vi "Find Zombies.vi"(8 "Error In":errorcluster) -> (0 "Error Out":errorcluster)   [LabVIEW 2018, in "Tests.lvlib" / "Toolkit.lvlib"]
uses:
  Toolkit.lvlib
  <vilib>/addons/_JKI Toolkits/Caraya/classes/Test/Test.lvclass
  <vilib>/addons/_JKI Toolkits/Caraya/classes/Assert/Assert.lvclass
  src/Toolkit/Toolkit.lvlib
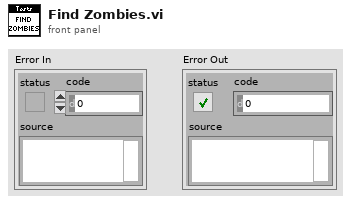
[diagram p1: front panel]
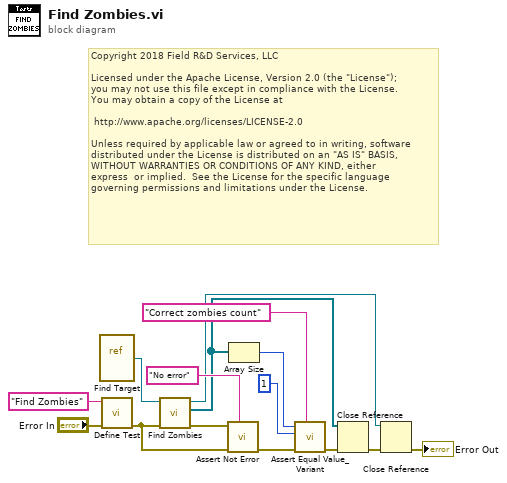
[diagram p0: block diagram]
diagram:
  # "Copyright 2018 Field R&D Services, LLC\n\nLicensed under the Apache License, Version 2.0 (the \"License\");\nyou may not use this file except in compliance with the License.\nYou may obtain a copy of the License at\n\n\thttp://www.apache.org/licenses/LICENSE-2.0\n\nUnless required by applicable law or agreed to in writing, software\ndistributed under the License is distributed on an \"AS IS\" BASIS,\nWITHOUT WARRANTIES OR CONDITIONS OF ANY KIND, either \nexpress  or implied.  See the License for the specific language \ngoverning permissions and limitations under the License."
  n1 = vi-ref "Find Target.vi"() -> (w6:refnum<vi>)
  n2 = call <vilib>:"Define Test.vi"("error in (no error)"="Error In", "Label (VI Title)"="Find Zombies") -> ("error out"=w5:errorcluster)  [unwired: 9 in]
  n3 = call "Find Zombies.vi"("Error In"=w5, "VI In"=w6) -> ("Error Out"=w15:errorcluster, "Graves"=w3:refnum<vi>[], "VI Out"=w7:refnum<vi>)  [unwired: 7 in]
  n4 = call <vilib>:"Assert Not Error.vi"("Label"="No error", "error in (no error)"=w5, "Not Error?"=w15) -> ("error out"=w12:errorcluster)  [unwired: 8 in]
  n5 = Array Size(array=w3) -> (size(s)=w2:i32)
  n6 = call <vilib>:"Assert Equal Value_Variant.vi"("Label"="Correct zombies count", "error in (no error)"=w12, "Y"=1 ("size(s)"), "X"=w2) -> ("error out"=w9:errorcluster)  [unwired: 7 in]
  n7 = Close Reference(reference=w3, error in (no error)=w9) -> (error out=w4:errorcluster)
  n8 = Close Reference(reference=w7, error in (no error)=w4) -> (error out=→"Error Out":errorcluster)
